vi "Read Command.vi"(7 "Addr":string="00", 11 "TEC Cmd":T1) -> (2 "String":string, 3 "Numeric":i32)   [LabVIEW 2015, in "TE Cooler.lvlib" / "TE Cooler.lvclass"]
uses:
  TE Cooler.lvclass
  Controls/Command.ctl
  Controls/Hex Cmd.ctl
  Controls/Scale IO.ctl
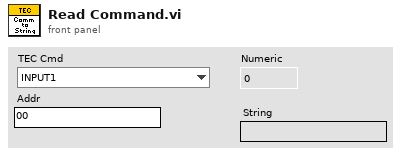
[diagram p1: front panel]
types:
  T1 = typedef "TE Cooler.lvlib/TE Cooler.lvclass/Command.ctl" = enum16{"INPUT1", "DESIRED CONTROL VALUE", "POWER OUTPUT", "ALARM STATUS", "INPUT 2", "OUTPUT CURRENT COUNTS", "ALARM TYPE", "SET TYPE DEFINE", "SENSOR TYPE", "CONTROL TYPE", "CONTROL OUTPUT POLARITY", "POWER ON/OFF", "OUTPUT SHUTDOWN IF ALARM", "FIXED DESIRED CONTROL SETTING", "PROPORTIONAL BANDWIDTH", "INTEGRAL GAIN", "DERIVATIVE GAIN", "LOW EXTERNAL SET RANGE", "HIGH EXTERNAL SET RANGE", "ALARM DEADBAND", "HIGH ALARM SETTING", "LOW ALARM SETTING", "CONTROL DEADBAND SETTING", "INPUT1 OFFSET", "INPUT2 OFFSET", "HEAT MULTIPLIER", "COOL MULTIPLIER", "OVER CURRENT COUNT COMPARE VALUE", "ALARM LATCH ENABLE", "NOT USED", "ALARM LATCH RESET", "CHOOSE SENSOR FOR ALARM FUNCTION", "CHOOSE TEMPERATURE WORKING UNITS", "EEPROM WRITE ENABLE", "OVER CURRENT CONTINUOUS", "OVER CURRENT RESTART ATTEMPTS", "JP3 DISPLAY ENABLE"}
  T2 = typedef "TE Cooler.lvlib/TE Cooler.lvclass/Scale IO.ctl" = i32[][]
  T3 = typedef "TE Cooler.lvlib/TE Cooler.lvclass/Hex Cmd.ctl" = string[][]
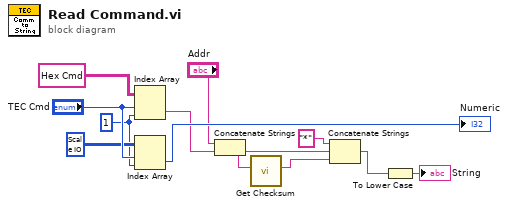
[diagram p0: block diagram]
diagram:
  w7 = 1 ("disabled index (col)")
  n1 = Index Array(array=T3 [["", "01"], ["", "03"], ["", "02"], ["", "05"], ["", "06"], ["", "07"], ["28", "41"], ["29", "42"], ["2a", "43"], ["2b", "44"], ["2c", "45"], ["2d", "46"], ["2e", "47"], ["1c", "50"], ["1d", "51"], ["1e", "52"], ["1f", "53"], ["20", "54"], ["21", "55"], ["22", "56"], ["23", "57"], ["24", "58"], ["25", "59"], ["26", "5a"], ["27", "5b"], ["0c", "5c"], ["0d", "5d"], ["0e", "5e"], ["2f", "48"], ["", ""], ["33", ""], ["31", "4a"], ["32", "4b"], ["34", "4c"], ["35", "4d"], ["0f", "5f"], ["36", "4e"]] ("Hex Cmd"), index (row)="TEC Cmd", index (col)=w7) -> (element=w5:string)
  n2 = Index Array(array=T2 [[0, 100], [0, 100], [0, 511], [0, 1], [0, 100], [0, 1], [1, 1], [1, 1], [1, 1], [1, 1], [1, 1], [1, 1], [100, 100], [100, 100], [100, 100], [100, 100], [1, 1], [1, 1], [100, 100], [100, 100], [100, 100], [100, 100], [100, 100], [100, 100], [100, 100], [100, 100], [100, 100], [1, 1], [1, 1], [0, 0], [1, 0], [1, 1], [1, 1], [1, 1], [1, 1], [1, 1], [1, 1]] ("Scale IO"), index (row)="TEC Cmd", index (col)=w7) -> (element=→"Numeric":i32)
  n3 = Concatenate Strings("Addr", w5) -> (w3:string)
  n4 = call "Get Checksum.vi"("Input"=w3) -> ("Checksum"=w4:string)  [unwired: 10 in]
  n5 = Concatenate Strings("*" ("string"), w3, w4) -> (w6:string)
  n6 = To Lower Case(string=w6) -> (all lower case string=→"String":string)
